vi "Convert Filter to INI String.vi"(11 "Filter Info":T1={"Filter Column"=enum."Description", "Filter Type"=enum."Contains", "Filter Value"="", "New Data?"=FALSE, "Enabled?"=FALSE}) -> (3 "INI String":string)   [LabVIEW 2023, in "VI Properties Editor.lvlib"]
doc: "Converts <B>Filter Info</B> to an INI string to be stored."
uses:
  VI Properties Editor.lvlib
  CTLs/Filter Info.ctl
  CTLs/Column Name.ctl
  CTLs/Filter Type.ctl
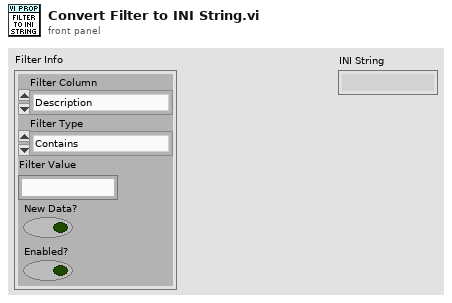
[diagram p1: front panel]
types:
  T1 = typedef "VI Properties Editor.lvlib/Filter Info.ctl" = cluster{"Filter Column":T2, "Filter Type":T3, "Filter Value":string, "New Data?":bool, "Enabled?":bool}
  T2 = typedef "VI Properties Editor.lvlib/Column Name.ctl" = enum16{"Name", "Path", "Type", "Window Title", "Description", "Help Path", "Help Tag", "Custom Title?", "Reentrant?", "Inlined?"}
  T3 = typedef "VI Properties Editor.lvlib/Filter Type.ctl" = enum16{"Contains", "Equals", "Starts with", "Ends with", "Does not contain", "Does not equal", "Is empty", "Is not empty"}
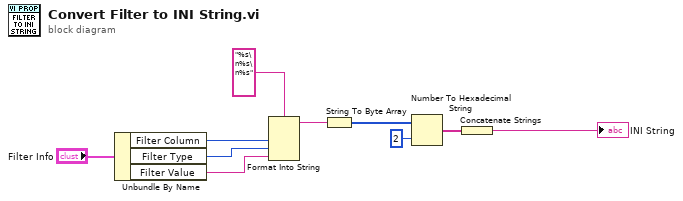
[diagram p0: block diagram]
diagram:
  n1 = Unbundle By Name("Filter Info") -> ("Filter Column"=w7:T2, "Filter Type"=w6:T3, "Filter Value"=w5:string)
  n2 = Format Into String(format string="%s\n%s\n%s", w7, w6, w5) -> (resulting string=w4:string)  [unwired: 2 in, 1 out]
  n3 = String To Byte Array(string=w4) -> (unsigned byte array=w9:u8[])
  n4 = Number To Hexadecimal String(1:i16 2 ("width (-)"), 2:w9) -> (0:w3:string[])
  n5 = Concatenate Strings(w3) -> (→"INI String":string)
